vi "Fetch Multi Eval Meas List ES Flatness Subcarrier Index Current Results.vi"(7 "Range (1)":T1=1, 8 "error in (no error)":errorcluster, 9 "Current Power (Minimum)":i32(ring) items=["Minimum", "Maximum"], 10 "Instance (1)":T2=1, 11 "VISA resource name":refnum<visa-resource-name>) -> (0 "error out":errorcluster, 1 "ES Flatness Subcarrier Results":dbl[](array[numeric]) format="%^.3e", 2 "Reliability":i32, 3 "VISA resource name out":refnum<visa-resource-name>)   [LabVIEW 2020, in "Rohde&Schwarz CMXP NR FR2 Measurement.lvlib"]
doc: "Returns subcarrier indices of the equalizer spectrum flatness measurement for all measured list mode segments.\n\nAttributes:\nRSCMXPNRFR2M_ATTR_FETCH_MULTI_EVAL_MEASUREMENT_LIST_ESF_SCINDEX_MAXIMUM_CURRENT_RESULTS\nRSCMXPNRFR2M_ATTR_FETCH_MULTI_EVAL_MEASUREMENT_LIST_ESF_SCINDEX_MINIMUM_CURRENT_RESULTS\n\nRemote-control commands:\nFETCh:NRMMw:MEAS<i>:MEValuation:LIST:ESFLatness:SCINdex:MAXimum<no>:CURRent?\nFETCh:NRMMw:MEAS<i>:MEValuation:LIST:ESFLatness:SCINdex:MINimum<no>:CURRent?"
uses:
  <instrlib>/Rohde&Schwarz CMXP NR FR2 Measurement/Rohde&Schwarz CMXP NR FR2 Measurement.lvlib
  <instrlib>/Rohde&Schwarz CMXP NR FR2 Measurement/Private/_Instance.ctl
  <instrlib>/Rohde&Schwarz CMXP NR FR2 Measurement/Private/_Range.ctl
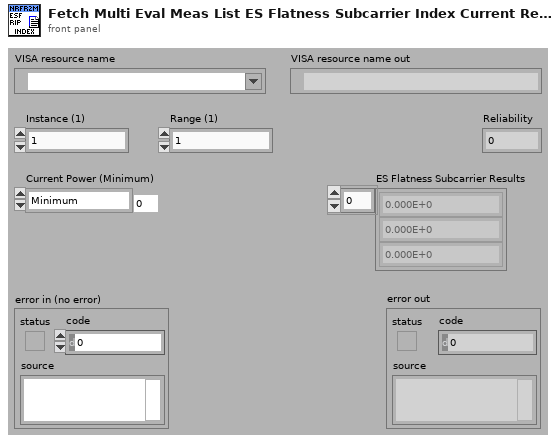
[diagram p1: front panel]
types:
  T1 = typedef "Rohde&Schwarz CMXP NR FR2 Measurement.lvlib/_Range.ctl" = i32
  T2 = typedef "Rohde&Schwarz CMXP NR FR2 Measurement.lvlib/_Instance.ctl" = i32
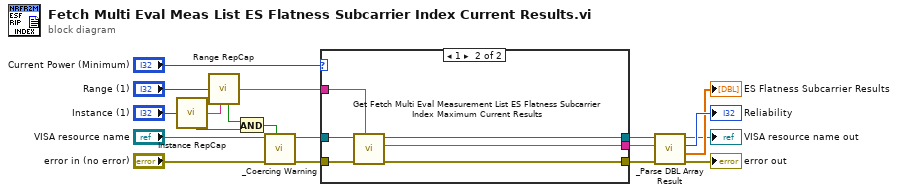
[diagram p0: block diagram]
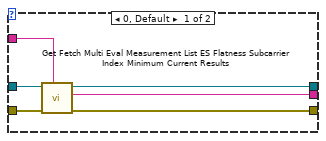
[diagram p2: hidden frame]
diagram:
  n1 = call <instrlib>:"Instance RepCap.vi"("Instance In"="Instance (1)") -> ("In Range?"=w17:bool, "RepCap Identifier Out"=w1:string)  [unwired: 1 in]
  n2 = call <instrlib>:"Range RepCap.vi"("Range In"="Range (1)", "RepCap String In (\"\")"=w1) -> ("In Range?"=w19:bool, "RepCap Identifier Out"=w13:string)
  n3 = And(x=w19, y=w17) -> (x .and. y?=w18:bool)
  n4 = call <instrlib>:"_Coercing Warning.vi"("In Range?"=w18, "error in (no error)"="error in (no error)", "VISA resource name"="VISA resource name") -> ("error out"=w12:errorcluster, "VISA resource name out"=w11:refnum<visa-resource-name>)  [unwired: 7 in]
  n5 = case shown="1" "Current Power (Minimum)" {
    tunnel: w13 -> [w25 w31]
    tunnel: w12 -> [w24 w30]
    tunnel: w11 -> [w23 w29]
    tunnel: [w22 w28] -> w9
    tunnel: [w21 w27] -> w8
    tunnel: [w20 w26] -> w7
    frame 0, Default {
      n6 = call "Get Fetch Multi Eval Measurement List ES Flatness Subcarrier Index Minimum Current Results"("Repeated Capabilities"=w25, "error in (no error)"=w24, "instrument handle"=w23) -> ("error out"=w22:errorcluster, "Fetch Multi Eval Measurement List ES Flatness Subcarrier Index Minimum Current Results"=w21:string, "instrument handle out"=w20:refnum<visa-resource-name>)  [unwired: 6 in]
    }
    frame 1 {
      n7 = call "Get Fetch Multi Eval Measurement List ES Flatness Subcarrier Index Maximum Current Results"("Repeated Capabilities"=w31, "error in (no error)"=w30, "instrument handle"=w29) -> ("error out"=w28:errorcluster, "Fetch Multi Eval Measurement List ES Flatness Subcarrier Index Maximum Current Results"=w27:string, "instrument handle out"=w26:refnum<visa-resource-name>)  [unwired: 6 in]
    }
  }
  n8 = call <instrlib>:"_Parse DBL Array Result.vi"("error in (no error)"=w9, "Input String"=w8, "VISA resource name"=w7) -> ("error out"=→"error out":errorcluster, "Results"=→"ES Flatness Subcarrier Results":dbl[], "Reliability"=→"Reliability":i32, "VISA resource name out"=→"VISA resource name out":refnum<visa-resource-name>)  [unwired: 5 in]
